vi "Error Report.vi"(8 "error in (no error)":errorcluster, 10 "Additional info":string, 11 "Error Code":i16) -> (0 "error out":errorcluster)   [LabVIEW 2018]
uses:
  <vilib>/Utility/error.llb/Error Cluster From Error Code.vi
  <vilib>/ErrorRing/Error Ring.xnode
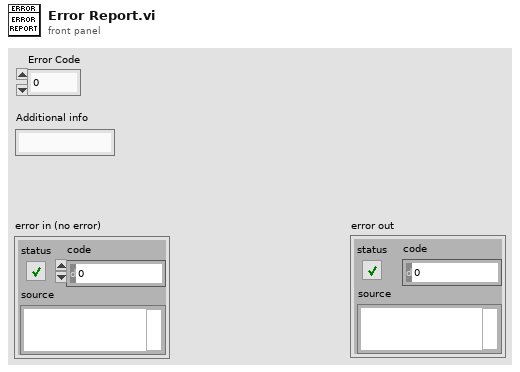
[diagram p1: front panel]
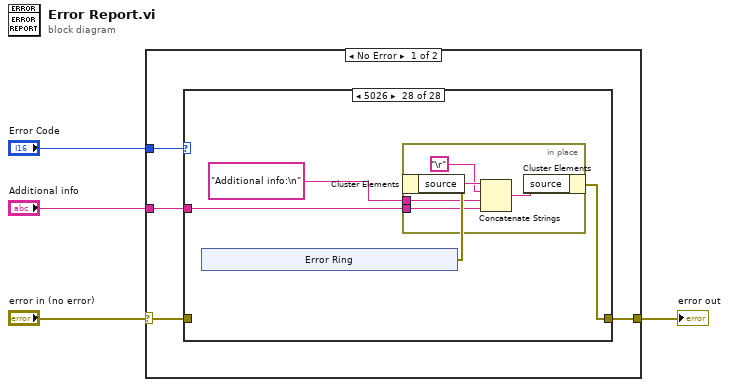
[diagram p0: block diagram]
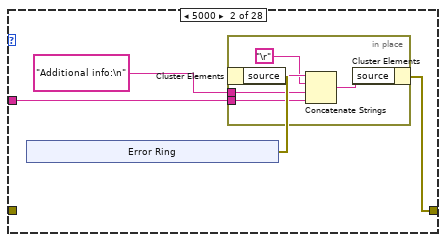
[diagram p3: hidden frame]
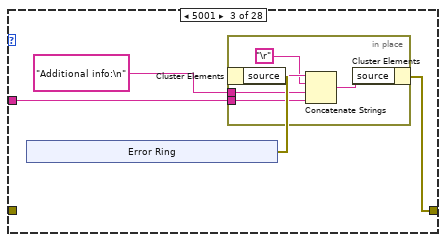
[diagram p4: hidden frame]
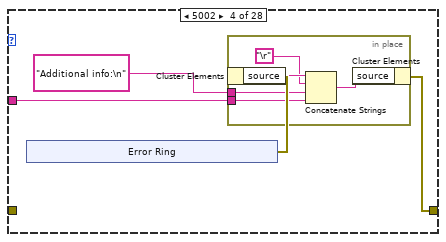
[diagram p5: hidden frame]
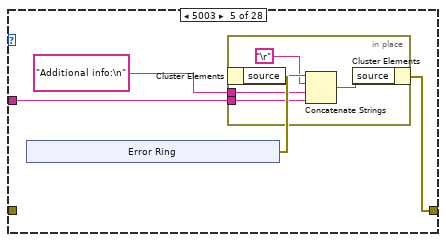
[diagram p6: hidden frame]
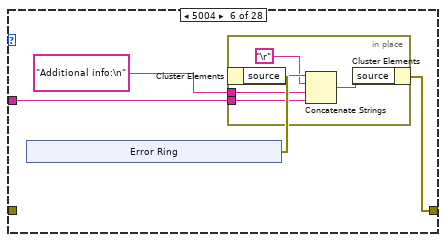
[diagram p7: hidden frame]
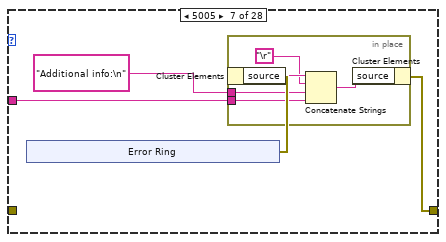
[diagram p8: hidden frame]
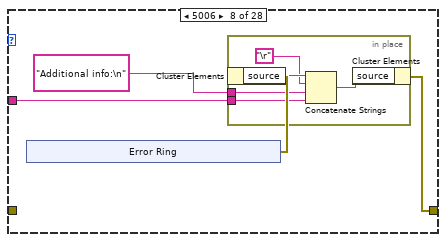
[diagram p9: hidden frame]
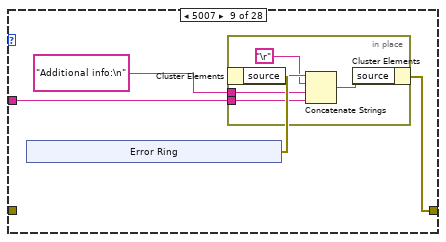
[diagram p10: hidden frame]
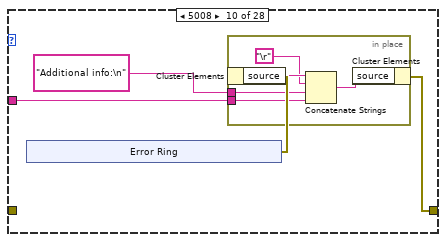
[diagram p11: hidden frame]
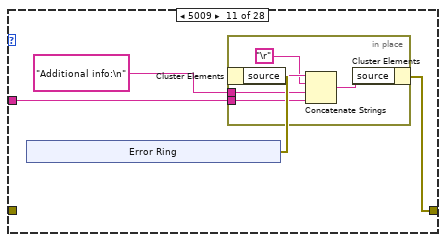
[diagram p12: hidden frame]
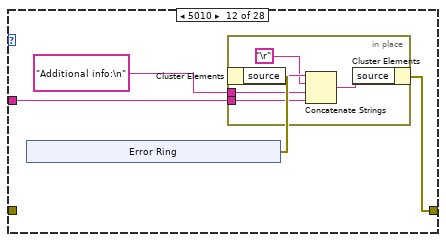
[diagram p13: hidden frame]
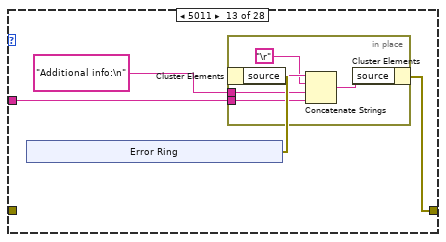
[diagram p14: hidden frame]
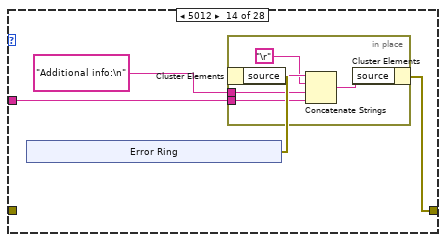
[diagram p15: hidden frame]
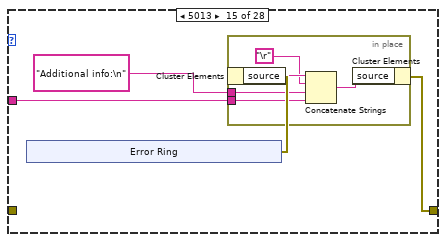
[diagram p16: hidden frame]
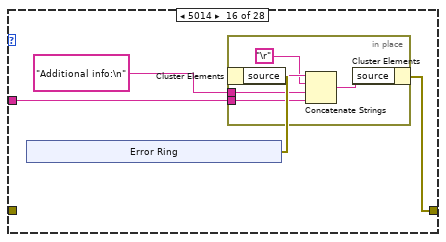
[diagram p17: hidden frame]
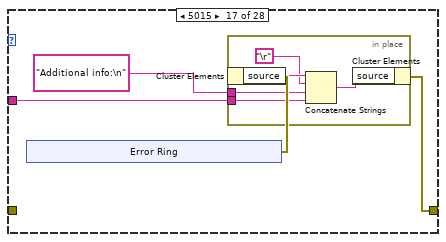
[diagram p18: hidden frame]
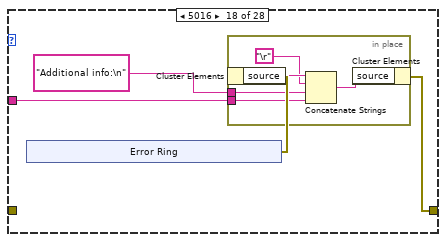
[diagram p19: hidden frame]
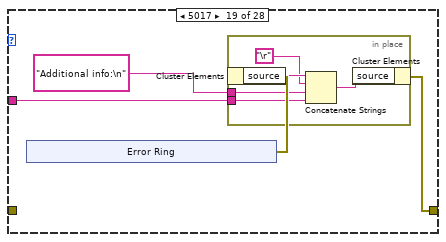
[diagram p20: hidden frame]
diagram:
  n1 = case shown="No Error" "error in (no error)" {
    selector: "error in (no error)" -> [w5 w388]
    tunnel: "Error Code" -> [w8 _]
    tunnel: "Additional info" -> [w7 _]
    tunnel: [w6 w388] -> w1
    frame No Error {
      n2 = case shown="5026" w8 {
        tunnel: w7 -> [_ w12 w26 w40 w54 w68 w82 w96 w110 w124 w138 w152 w166 w180 w194 w208 w222 w236 w250 w264 w278 w292 w306 w320 w334 w348 w362 w376]
        tunnel: [w9 w10 w24 w38 w52 w66 w80 w94 w108 w122 w136 w150 w164 w178 w192 w206 w220 w234 w248 w262 w276 w290 w304 w318 w332 w346 w360 w374] -> w6
        tunnel: w5 -> [w9 _ _ _ _ _ _ _ _ _ _ _ _ _ _ _ _ _ _ _ _ _ _ _ _ _ _ _]
        frame 0, Default {
        }
        frame 5000 {
          n3 = xnode "Error Ring"() -> ("error out"=w13:errorcluster)
          n4 = in-place {
            in-place-border: w12 -> [w15]
            in-place-border: "Additional info:\n" ("Additional info") -> [w16]
            n5 = in-place-cluster #1(w13) -> ("source"=w18:string)
            n6 = Concatenate Strings(w18, "\r", w16, w15) -> (w14:string)
            n7 = in-place-cluster #1("source"=w14) -> (w10:errorcluster)
          }
        }
        frame 5001 {
          n8 = xnode "Error Ring"() -> ("error out"=w27:errorcluster)
          n9 = in-place {
            in-place-border: w26 -> [w29]
            in-place-border: "Additional info:\n" ("Additional info") -> [w30]
            n10 = in-place-cluster #2(w27) -> ("source"=w32:string)
            n11 = Concatenate Strings(w32, "\r", w30, w29) -> (w28:string)
            n12 = in-place-cluster #2("source"=w28) -> (w24:errorcluster)
          }
        }
        frame 5002 {
          n13 = xnode "Error Ring"() -> ("error out"=w41:errorcluster)
          n14 = in-place {
            in-place-border: w40 -> [w43]
            in-place-border: "Additional info:\n" ("Additional info") -> [w44]
            n15 = in-place-cluster #3(w41) -> ("source"=w46:string)
            n16 = Concatenate Strings(w46, "\r", w44, w43) -> (w42:string)
            n17 = in-place-cluster #3("source"=w42) -> (w38:errorcluster)
          }
        }
        frame 5003 {
          n18 = xnode "Error Ring"() -> ("error out"=w55:errorcluster)
          n19 = in-place {
            in-place-border: w54 -> [w57]
            in-place-border: "Additional info:\n" ("Additional info") -> [w58]
            n20 = in-place-cluster #4(w55) -> ("source"=w60:string)
            n21 = Concatenate Strings(w60, "\r", w58, w57) -> (w56:string)
            n22 = in-place-cluster #4("source"=w56) -> (w52:errorcluster)
          }
        }
        frame 5004 {
          n23 = xnode "Error Ring"() -> ("error out"=w69:errorcluster)
          n24 = in-place {
            in-place-border: w68 -> [w71]
            in-place-border: "Additional info:\n" ("Additional info") -> [w72]
            n25 = in-place-cluster #5(w69) -> ("source"=w74:string)
            n26 = Concatenate Strings(w74, "\r", w72, w71) -> (w70:string)
            n27 = in-place-cluster #5("source"=w70) -> (w66:errorcluster)
          }
        }
        frame 5005 {
          n28 = xnode "Error Ring"() -> ("error out"=w83:errorcluster)
          n29 = in-place {
            in-place-border: w82 -> [w85]
            in-place-border: "Additional info:\n" ("Additional info") -> [w86]
            n30 = in-place-cluster #6(w83) -> ("source"=w88:string)
            n31 = Concatenate Strings(w88, "\r", w86, w85) -> (w84:string)
            n32 = in-place-cluster #6("source"=w84) -> (w80:errorcluster)
          }
        }
        frame 5006 {
          n33 = xnode "Error Ring"() -> ("error out"=w97:errorcluster)
          n34 = in-place {
            in-place-border: w96 -> [w99]
            in-place-border: "Additional info:\n" ("Additional info") -> [w100]
            n35 = in-place-cluster #7(w97) -> ("source"=w102:string)
            n36 = Concatenate Strings(w102, "\r", w100, w99) -> (w98:string)
            n37 = in-place-cluster #7("source"=w98) -> (w94:errorcluster)
          }
        }
        frame 5007 {
          n38 = xnode "Error Ring"() -> ("error out"=w111:errorcluster)
          n39 = in-place {
            in-place-border: w110 -> [w113]
            in-place-border: "Additional info:\n" ("Additional info") -> [w114]
            n40 = in-place-cluster #8(w111) -> ("source"=w116:string)
            n41 = Concatenate Strings(w116, "\r", w114, w113) -> (w112:string)
            n42 = in-place-cluster #8("source"=w112) -> (w108:errorcluster)
          }
        }
        frame 5008 {
          n43 = xnode "Error Ring"() -> ("error out"=w125:errorcluster)
          n44 = in-place {
            in-place-border: w124 -> [w127]
            in-place-border: "Additional info:\n" ("Additional info") -> [w128]
            n45 = in-place-cluster #9(w125) -> ("source"=w130:string)
            n46 = Concatenate Strings(w130, "\r", w128, w127) -> (w126:string)
            n47 = in-place-cluster #9("source"=w126) -> (w122:errorcluster)
          }
        }
        frame 5009 {
          n48 = xnode "Error Ring"() -> ("error out"=w139:errorcluster)
          n49 = in-place {
            in-place-border: w138 -> [w141]
            in-place-border: "Additional info:\n" ("Additional info") -> [w142]
            n50 = in-place-cluster #10(w139) -> ("source"=w144:string)
            n51 = Concatenate Strings(w144, "\r", w142, w141) -> (w140:string)
            n52 = in-place-cluster #10("source"=w140) -> (w136:errorcluster)
          }
        }
        frame 5010 {
          n53 = xnode "Error Ring"() -> ("error out"=w153:errorcluster)
          n54 = in-place {
            in-place-border: w152 -> [w155]
            in-place-border: "Additional info:\n" ("Additional info") -> [w156]
            n55 = in-place-cluster #11(w153) -> ("source"=w158:string)
            n56 = Concatenate Strings(w158, "\r", w156, w155) -> (w154:string)
            n57 = in-place-cluster #11("source"=w154) -> (w150:errorcluster)
          }
        }
        frame 5011 {
          n58 = xnode "Error Ring"() -> ("error out"=w167:errorcluster)
          n59 = in-place {
            in-place-border: w166 -> [w169]
            in-place-border: "Additional info:\n" ("Additional info") -> [w170]
            n60 = in-place-cluster #12(w167) -> ("source"=w172:string)
            n61 = Concatenate Strings(w172, "\r", w170, w169) -> (w168:string)
            n62 = in-place-cluster #12("source"=w168) -> (w164:errorcluster)
          }
        }
        frame 5012 {
          n63 = xnode "Error Ring"() -> ("error out"=w181:errorcluster)
          n64 = in-place {
            in-place-border: w180 -> [w183]
            in-place-border: "Additional info:\n" ("Additional info") -> [w184]
            n65 = in-place-cluster #13(w181) -> ("source"=w186:string)
            n66 = Concatenate Strings(w186, "\r", w184, w183) -> (w182:string)
            n67 = in-place-cluster #13("source"=w182) -> (w178:errorcluster)
          }
        }
        frame 5013 {
          n68 = xnode "Error Ring"() -> ("error out"=w195:errorcluster)
          n69 = in-place {
            in-place-border: w194 -> [w197]
            in-place-border: "Additional info:\n" ("Additional info") -> [w198]
            n70 = in-place-cluster #14(w195) -> ("source"=w200:string)
            n71 = Concatenate Strings(w200, "\r", w198, w197) -> (w196:string)
            n72 = in-place-cluster #14("source"=w196) -> (w192:errorcluster)
          }
        }
        frame 5014 {
          n73 = xnode "Error Ring"() -> ("error out"=w209:errorcluster)
          n74 = in-place {
            in-place-border: w208 -> [w211]
            in-place-border: "Additional info:\n" ("Additional info") -> [w212]
            n75 = in-place-cluster #15(w209) -> ("source"=w214:string)
            n76 = Concatenate Strings(w214, "\r", w212, w211) -> (w210:string)
            n77 = in-place-cluster #15("source"=w210) -> (w206:errorcluster)
          }
        }
        frame 5015 {
          n78 = xnode "Error Ring"() -> ("error out"=w223:errorcluster)
          n79 = in-place {
            in-place-border: w222 -> [w225]
            in-place-border: "Additional info:\n" ("Additional info") -> [w226]
            n80 = in-place-cluster #16(w223) -> ("source"=w228:string)
            n81 = Concatenate Strings(w228, "\r", w226, w225) -> (w224:string)
            n82 = in-place-cluster #16("source"=w224) -> (w220:errorcluster)
          }
        }
        frame 5016 {
          n83 = xnode "Error Ring"() -> ("error out"=w237:errorcluster)
          n84 = in-place {
            in-place-border: w236 -> [w239]
            in-place-border: "Additional info:\n" ("Additional info") -> [w240]
            n85 = in-place-cluster #17(w237) -> ("source"=w242:string)
            n86 = Concatenate Strings(w242, "\r", w240, w239) -> (w238:string)
            n87 = in-place-cluster #17("source"=w238) -> (w234:errorcluster)
          }
        }
        frame 5017 {
          n88 = xnode "Error Ring"() -> ("error out"=w251:errorcluster)
          n89 = in-place {
            in-place-border: w250 -> [w253]
            in-place-border: "Additional info:\n" ("Additional info") -> [w254]
            n90 = in-place-cluster #18(w251) -> ("source"=w256:string)
            n91 = Concatenate Strings(w256, "\r", w254, w253) -> (w252:string)
            n92 = in-place-cluster #18("source"=w252) -> (w248:errorcluster)
          }
        }
        frame 5018 {
          n93 = xnode "Error Ring"() -> ("error out"=w265:errorcluster)
          n94 = in-place {
            in-place-border: w264 -> [w267]
            in-place-border: "Additional info:\n" ("Additional info") -> [w268]
            n95 = in-place-cluster #19(w265) -> ("source"=w270:string)
            n96 = Concatenate Strings(w270, "\r", w268, w267) -> (w266:string)
            n97 = in-place-cluster #19("source"=w266) -> (w262:errorcluster)
          }
        }
        frame 5019 {
          n98 = xnode "Error Ring"() -> ("error out"=w279:errorcluster)
          n99 = in-place {
            in-place-border: w278 -> [w281]
            in-place-border: "Additional info:\n" ("Additional info") -> [w282]
            n100 = in-place-cluster #20(w279) -> ("source"=w284:string)
            n101 = Concatenate Strings(w284, "\r", w282, w281) -> (w280:string)
            n102 = in-place-cluster #20("source"=w280) -> (w276:errorcluster)
          }
        }
        frame 5020 {
          n103 = xnode "Error Ring"() -> ("error out"=w293:errorcluster)
          n104 = in-place {
            in-place-border: w292 -> [w295]
            in-place-border: "Additional info:\n" ("Additional info") -> [w296]
            n105 = in-place-cluster #21(w293) -> ("source"=w298:string)
            n106 = Concatenate Strings(w298, "\r", w296, w295) -> (w294:string)
            n107 = in-place-cluster #21("source"=w294) -> (w290:errorcluster)
          }
        }
        frame 5021 {
          n108 = xnode "Error Ring"() -> ("error out"=w307:errorcluster)
          n109 = in-place {
            in-place-border: w306 -> [w309]
            in-place-border: "Additional info:\n" ("Additional info") -> [w310]
            n110 = in-place-cluster #22(w307) -> ("source"=w312:string)
            n111 = Concatenate Strings(w312, "\r", w310, w309) -> (w308:string)
            n112 = in-place-cluster #22("source"=w308) -> (w304:errorcluster)
          }
        }
        frame 5022 {
          n113 = xnode "Error Ring"() -> ("error out"=w321:errorcluster)
          n114 = in-place {
            in-place-border: w320 -> [w323]
            in-place-border: "Additional info:\n" ("Additional info") -> [w324]
            n115 = in-place-cluster #23(w321) -> ("source"=w326:string)
            n116 = Concatenate Strings(w326, "\r", w324, w323) -> (w322:string)
            n117 = in-place-cluster #23("source"=w322) -> (w318:errorcluster)
          }
        }
        frame 5023 {
          n118 = xnode "Error Ring"() -> ("error out"=w335:errorcluster)
          n119 = in-place {
            in-place-border: w334 -> [w337]
            in-place-border: "Additional info:\n" ("Additional info") -> [w338]
            n120 = in-place-cluster #24(w335) -> ("source"=w340:string)
            n121 = Concatenate Strings(w340, "\r", w338, w337) -> (w336:string)
            n122 = in-place-cluster #24("source"=w336) -> (w332:errorcluster)
          }
        }
        frame 5024 {
          n123 = xnode "Error Ring"() -> ("error out"=w349:errorcluster)
          n124 = in-place {
            in-place-border: w348 -> [w351]
            in-place-border: "Additional info:\n" ("Additional info") -> [w352]
            n125 = in-place-cluster #25(w349) -> ("source"=w354:string)
            n126 = Concatenate Strings(w354, "\r", w352, w351) -> (w350:string)
            n127 = in-place-cluster #25("source"=w350) -> (w346:errorcluster)
          }
        }
        frame 5025 {
          n128 = xnode "Error Ring"() -> ("error out"=w363:errorcluster)
          n129 = in-place {
            in-place-border: w362 -> [w365]
            in-place-border: "Additional info:\n" ("Additional info") -> [w366]
            n130 = in-place-cluster #26(w363) -> ("source"=w368:string)
            n131 = Concatenate Strings(w368, "\r", w366, w365) -> (w364:string)
            n132 = in-place-cluster #26("source"=w364) -> (w360:errorcluster)
          }
        }
        frame 5026 {
          n133 = xnode "Error Ring"() -> ("error out"=w377:errorcluster)
          n134 = in-place {
            in-place-border: w376 -> [w379]
            in-place-border: "Additional info:\n" ("Additional info") -> [w380]
            n135 = in-place-cluster #27(w377) -> ("source"=w382:string)
            n136 = Concatenate Strings(w382, "\r", w380, w379) -> (w378:string)
            n137 = in-place-cluster #27("source"=w378) -> (w374:errorcluster)
          }
        }
      }
    }
    frame Error {
    }
  }
  "error out" <- w1
